vi "calculate_eqe.vi"(7 "Application Directory":string, 9 "wavelengths":dbl[](array[numeric]), 10 "current measurements":dbl[](array[numeric]), 11 "Ref data filepath":path) -> (2 "eqe measurements":dbl[](array[numeric]))   [LabVIEW 2016]
uses:
  <vilib>/Utility/file.llb/Read Delimited Spreadsheet (DBL).vi
  <vilib>/gmath/NI_Gmath.lvlib
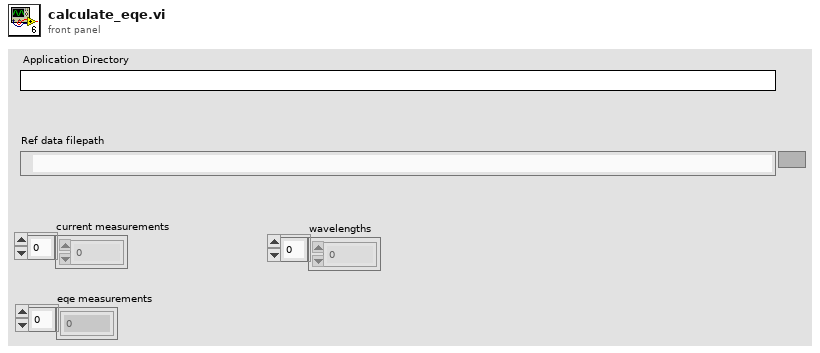
[diagram p1: front panel]
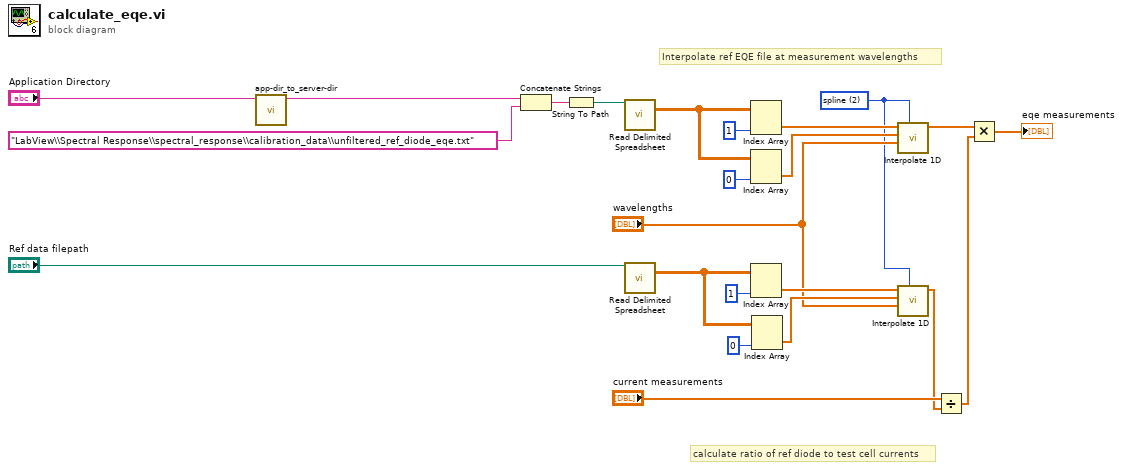
[diagram p0: block diagram]
diagram:
  w2 = 2 items=["nearest", "linear", "spline", "cubic Hermite", "Lagrange"] ("method")
  # "calculate ratio of ref diode to test cell currents"
  # "Interpolate ref EQE file at measurement wavelengths"
  n1 = call "app-dir_to_server-dir.vi"("Application Directory"="Application Directory") -> ("Group Server Directory"=w10:string)  [unwired: 10 in]
  n2 = Concatenate Strings(w10, "LabView\\Spectral Response\\spectral_response\\calibration_data\\unfiltered_ref_diode_eqe.txt" ("string")) -> (w8:string)
  n3 = String To Path(string=w8) -> (path=w11:path)
  n4 = call-poly <vilib>:"Read Delimited Spreadsheet.vi"("file path (dialog if empty)"=w11) -> ("all rows"=w16:dbl[][])  [unwired: 9 in, 5 out]
  n5 = call-poly <vilib>:"Read Delimited Spreadsheet.vi"("file path (dialog if empty)"="Ref data filepath") -> ("all rows"=w7:dbl[][])  [unwired: 9 in, 5 out]
  n6 = Index Array(array=w16, index (col)=1 ("disabled index (col)")) -> (element=w15:dbl[])  [unwired: 1 in]
  n7 = Index Array(array=w16, index (col)=0 ("disabled index (col)")) -> (element=w14:dbl[])  [unwired: 1 in]
  n8 = Index Array(array=w7, index (col)=1 ("disabled index (col)")) -> (element=w5:dbl[])  [unwired: 1 in]
  n9 = Index Array(array=w7, index (col)=0 ("index")) -> (element=w4:dbl[])  [unwired: 1 in]
  n10 = call <vilib>:"Interpolate 1D.vi"("method"=w2, "xi"="wavelengths", "X"=w14, "Y"=w15) -> ("yi"=w13:dbl[])  [unwired: 5 in, 2 out]
  n11 = call <vilib>:"Interpolate 1D.vi"("method"=w2, "xi"="wavelengths", "X"=w4, "Y"=w5) -> ("yi"=w1:dbl[])  [unwired: 5 in, 2 out]
  n12 = Divide(x="current measurements", y=w1) -> (x/y=w19:dbl[])
  n13 = Multiply(x=w13, y=w19) -> (x*y=→"eqe measurements":dbl[])
